vi "Initialize Attributes.vi"(8 "error in (no error)":errorcluster, 10 "Attribute Data":variant, 11 "CS++Syslog in":refnum<class "CS++Syslog.lvclass">) -> (0 "error out":errorcluster, 2 "Found?":bool, 3 "CS++Syslog out":refnum<class "CS++Syslog.lvclass">)   [LabVIEW 2014, in "CS++Syslog.lvlib" / "CS++Syslog.lvclass"]
doc: "Initialize object attribute.\n\nUnique resources should be allocated elsewhere!"
uses:
  CS++Syslog.lvclass
  CS++Syslog.lvclass/CS++Syslog.ctl
  CSPP_Core/Classes/CS++BaseClasses/MessageLogger/CS++MessageLogger.lvclass
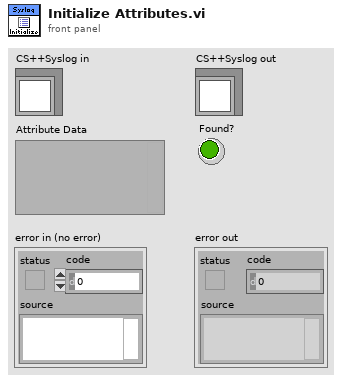
[diagram p1: front panel]
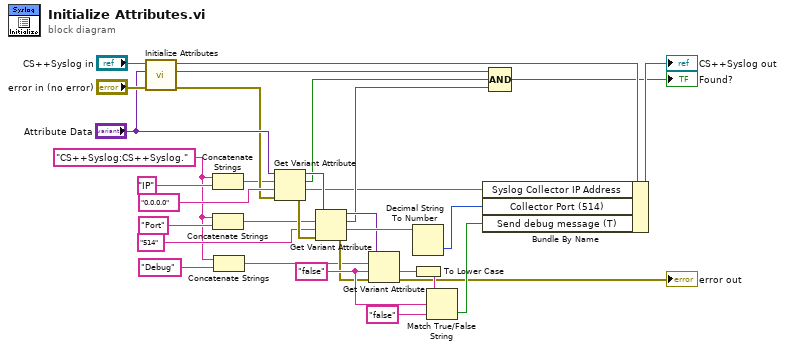
[diagram p0: block diagram]
diagram:
  w24 = "false" ("name")
  w1 = "CS++Syslog:CS++Syslog." ("name")
  n1 = call-parent "Initialize Attributes.vi"("error in (no error)"="error in (no error)", "Attribute Data"="Attribute Data", "CS++Base in"="CS++Syslog in") -> ("error out"=w11:errorcluster, "Found?"=w28:bool, "CS++Base out"=w30:refnum<class "CS++Syslog.lvclass">)  [unwired: 6 in]
  n2 = Concatenate Strings(w1, "IP" ("name")) -> (w4:string)
  n3 = Concatenate Strings(w1, "Port" ("name")) -> (w3:string)
  n4 = Concatenate Strings(w1, "Debug" ("name")) -> (w2:string)
  n5 = Get Variant Attribute(Variant="Attribute Data", name=w4, default value (empty Variant)="0.0.0.0" ("name"), error in=w11) -> (duplicate Variant=w16:variant, found=w10:bool, value=w6:string, error out=w18:errorcluster)
  n6 = Get Variant Attribute(Variant=w16, name=w3, default value (empty Variant)="514" ("Collector Port (514)"), error in=w18) -> (duplicate Variant=w19:variant, found=w9:bool, value=w22:string, error out=w20:errorcluster)
  n7 = Get Variant Attribute(Variant=w19, name=w2, default value (empty Variant)=w24, error in=w20) -> (value=w26:string, error out=→"error out":errorcluster)  [unwired: 2 out]
  n8 = Decimal String To Number(string=w22) -> (number=w7:i32)  [unwired: 2 in, 1 out]
  n9 = To Lower Case(string=w26) -> (all lower case string=w23:string)
  n10 = Match True/False String(2:"false" ("true string"), 3:w24, 4:w23) -> (0:w8:bool)  [unwired: 1 out]
  n11 = Bundle By Name(cluster=w30, "Syslog Collector IP Address"=w6, "Collector Port (514)"=w7, "Send debug message (T)"=w8) -> (→"CS++Syslog out":refnum<class "CS++Syslog.lvclass">)
  n12 = Compound Arithmetic op=AND(w28, w10, w9) -> (→"Found?":bool)
